vi "Edit Data Interactively.vi"(8 "error in (no error)":errorcluster, 11 "Attribute in":refnum<class "Attribute.lvclass">) -> (0 "error out":errorcluster, 2 "Cancel?":bool, 3 "Attribute out":refnum<class "Attribute.lvclass">)   [LabVIEW 2026, in "VILab.lvlib" / "Attribute.lvclass"]
uses:
  Attribute.lvclass
  Attribute.lvclass/Attribute.ctl
  Data Item/Data Item.lvclass
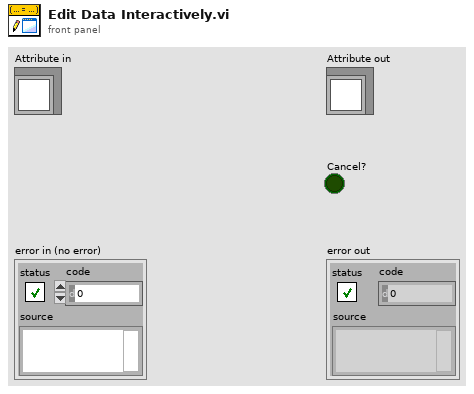
[diagram p1: front panel]
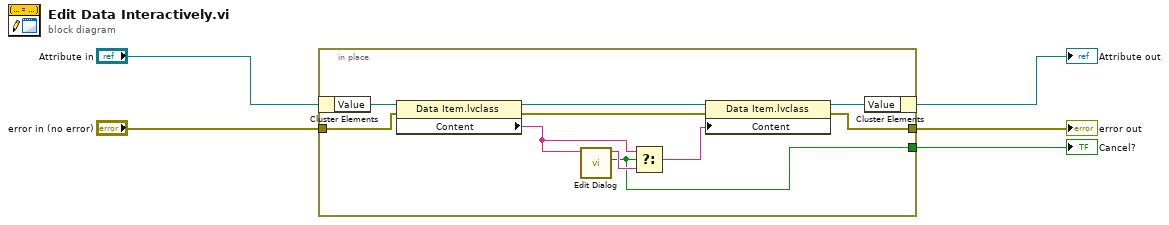
[diagram p0: block diagram]
diagram:
  n1 = in-place {
    in-place-border: "error in (no error)" -> [w6]
    in-place-border: [w8] -> w5
    in-place-border: [w12] -> w4
    n2 = in-place-cluster #1("Attribute in") -> ("Value"=w15:refnum<class "Data Item.lvclass">)
    n3 = property class="Data Item.lvclass"(reference=w15, error in=w6) -> (reference out=w11:refnum<class "Data Item.lvclass">, error out=w7:errorcluster, "Content"=w13:string)
    n4 = call "Edit Dialog.vi"("Content"=w13) -> ("Canceled?"=w12:bool, "String"=w14:string)  [unwired: 9 in]
    n5 = Select(t=w13, s=w12, f=w14) -> (s? t:f=w10:string)
    n6 = property class="Data Item.lvclass"(reference=w11, error in=w7, "Content"=w10) -> (reference out=w9:refnum<class "Data Item.lvclass">, error out=w8:errorcluster)
    n7 = in-place-cluster #1("Value"=w9) -> (→"Attribute out":refnum<class "Attribute.lvclass">)
  }
  "error out" <- w5
  "Cancel?" <- w4
